vi "saveSequence.vi"(0 "object in":refnum<class "Hamamatsu.lvclass">, 2 "folder path":path, 5 "error in (no error)":errorcluster) -> (14 "object out":refnum<class "Hamamatsu.lvclass">, 16 "Timestamps":dbl[](array[numeric]), 17 "Filenames":path[](array[path]), 19 "error out":errorcluster)   [LabVIEW 2024, in "Hamamatsu.lvclass"]
uses:
  Hamamatsu.lvclass
  Hamamatsu.lvclass/Hamamatsu.ctl
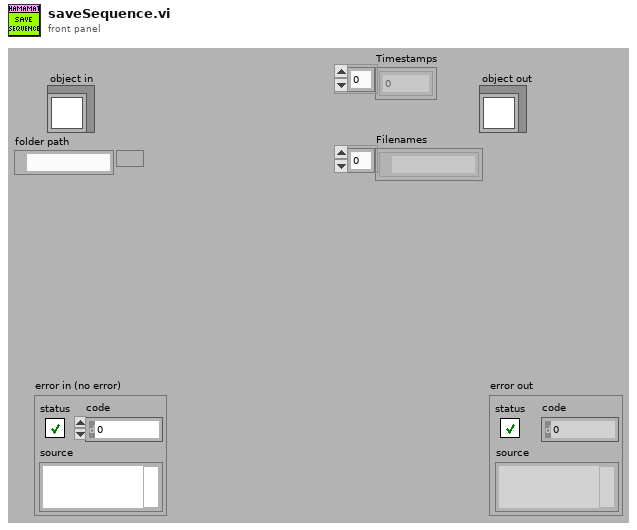
[diagram p1: front panel]
types:
  T1 = typedef "Image Type" = u32
  T2 = typedef "IMAQ Image.ctl" = refnum<image>
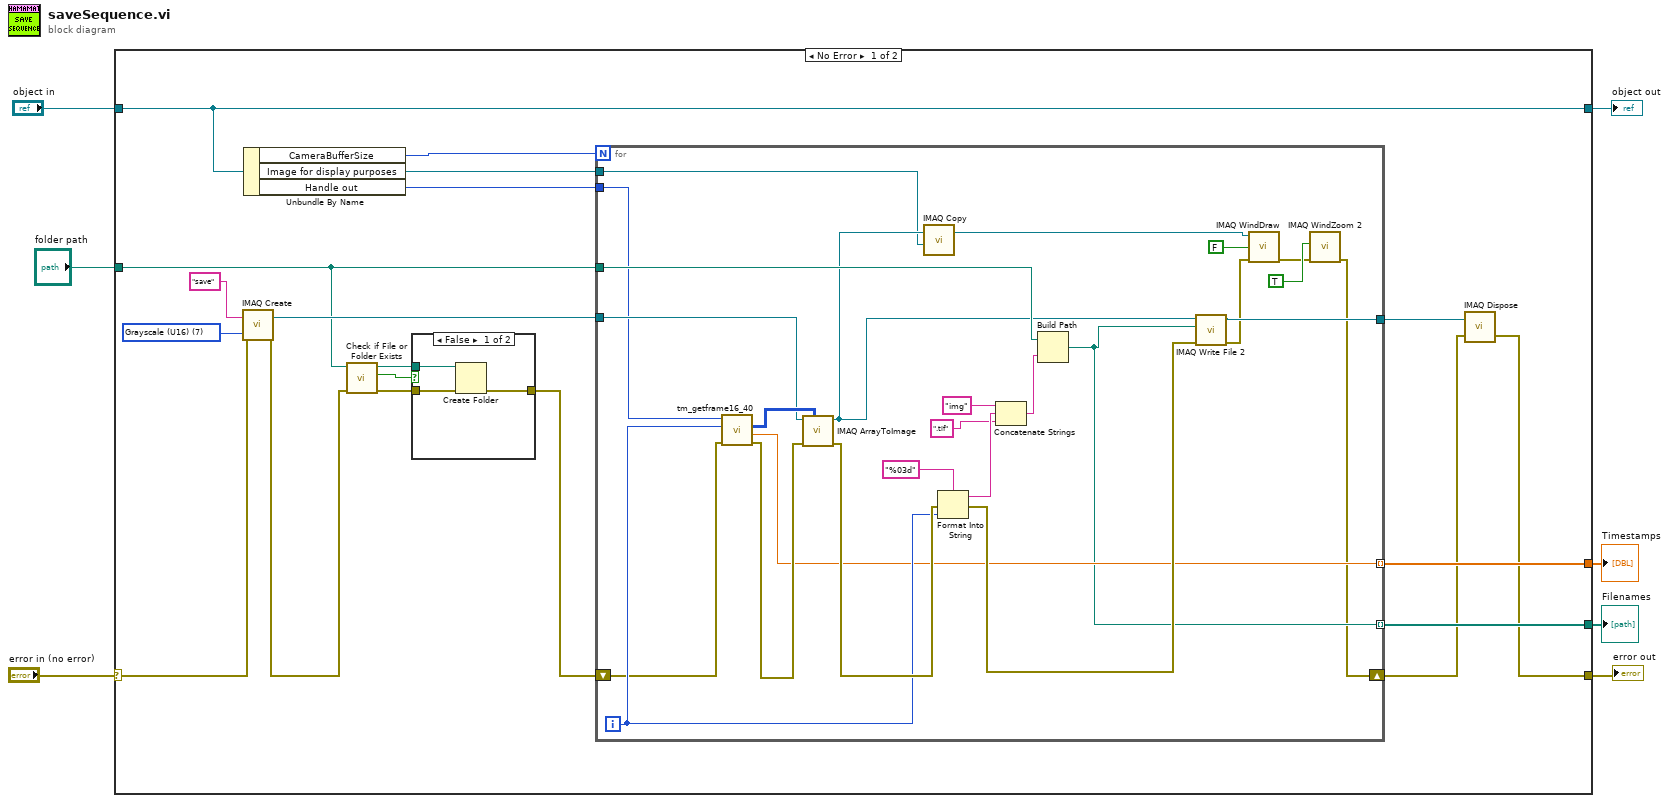
[diagram p0: block diagram]
diagram:
  n1 = case shown="No Error" "error in (no error)" {
    selector: "error in (no error)" -> [w21 w57]
    tunnel: [w16 w57] -> w6
    tunnel: [w26 w56] -> w4
    tunnel: "object in" -> [w26 w56]
    tunnel: "folder path" -> [w15 _]
    tunnel: [w20 _] -> w2
    tunnel: [w19 _] -> w1
    frame No Error {
      w22 = T1 7 items=["Grayscale (U8)", "Grayscale (I16)", "Grayscale (SGL)", "Complex (CSG)", "RGB (U32)", "HSL (U32)", "RGB (U64)", "Grayscale (U16)"] ("Image Type")
      n2 = call "IMAQ Create"("Image Name"="save", "Image Type"=w22, "error in (no error)"=w21) -> ("New Image"=w23:T2, "error out"=w13:errorcluster)  [unwired: 2 in]
      n3 = Unbundle By Name(w26) -> ("CameraBufferSize"=w25:i32, "Image for display purposes"=w9:T2, "Handle out"=w8:u32)
      n4 = call <vilib>:"Check if File or Folder Exists.vi"("error in (no error)"=w13, "path"=w15) -> ("error out"=w11:errorcluster, "file or folder exists?"=w12:bool, "dup path"=w14:path)  [unwired: 7 in]
      n5 = case shown="False" w12 {
        tunnel: w14 -> [w29 _]
        tunnel: w11 -> [w28 w30]
        tunnel: [w27 w30] -> w10
        frame False {
          n6 = Create Folder(path (use dialog)=w29, error in=w28) -> (error out=w27:errorcluster)  [unwired: 1 in, 2 out]
        }
        frame True {
        }
      }
      n7 = for {
        N: w25 -> [_]
        tunnel: w23 -> [w47]
        tunnel: w15 -> [w49]
        shift-right: [w32] -> w17
        shift-left: w10 -> [w44]
        tunnel: [w42] -> w20 mode=indexing
        tunnel: [w41] -> w19 mode=indexing
        tunnel: [w40] -> w18
        tunnel: w9 -> [w35]
        tunnel: w8 -> [w31]
        i -> [w45]
        n8 = call <userlib>:"tm_getframe16_40.vi"("error in (no error)"=w44, "Frame Index"=w45, "Handle in"=w31) -> ("error out"=w43:errorcluster, "Timestamp"=w42:dbl, "Data"=w48:u16[][])  [unwired: 5 in, 1 out]
        n9 = call "IMAQ ArrayToImage"("Image Pixels (U16)"=w48, "error in (no error)"=w43, "Image"=w47) -> ("error out"=w46:errorcluster, "Image Out"=w36:T2)  [unwired: 7 in]
        n10 = call "IMAQ Copy"("Image Dst"=w35, "Image Src"=w36) -> ("Image Dst Out"=w34:T2)  [unwired: 4 in, 1 out]
        n11 = Format Into String(format string="%03d", error in=w46, w45) -> (resulting string=w53:string, error out=w51:errorcluster)  [unwired: 1 in]
        n12 = Concatenate Strings("img" ("string"), w53, ".tif" ("string")) -> (w52:string)
        n13 = Build Path(base path=w49, name or relative path=w52) -> (appended path=w41:path)
        n14 = call-poly "IMAQ Write File 2"("error in (no error)"=w51, "File Path"=w41, "Image"=w36) -> ("error out"=w33:errorcluster, "Image Out (duplicate)"=w40:T2)  [unwired: 7 in]
        n15 = call "IMAQ WindDraw"("Resize to Image Size? (Y)"=FALSE, "error in (no error)"=w33, "Image"=w34) -> ("error out"=w37:errorcluster)  [unwired: 7 in, 1 out]
        n16 = call "IMAQ WindZoom 2"("error in (no error)"=w37, "Zoom to Fit? (False)"=TRUE) -> ("error out"=w32:errorcluster)  [unwired: 6 in, 3 out]
      }
      n17 = call "IMAQ Dispose"("Image"=w18, "error in (no error)"=w17) -> ("error out"=w16:errorcluster)  [unwired: 4 in]
    }
    frame Error {
    }
  }
  "error out" <- w6
  "object out" <- w4
  "Timestamps" <- w2
  "Filenames" <- w1
